vi "SetDacSafe2.vi"(1 "New Value (mV)":sgl format="%.2f", 2 "Actual Value DAC (mV)":dbl=299.98779296875 format="%.2f", 3 "DAC Nr.":i32=3 min=1 max=8 step=1) -> (0 "Voltage (mV) 2":sgl format="%.4f")   [LabVIEW 2011]
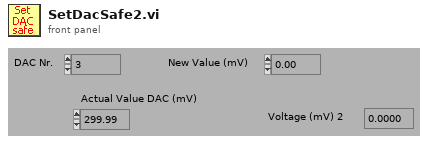
[diagram p1: front panel]
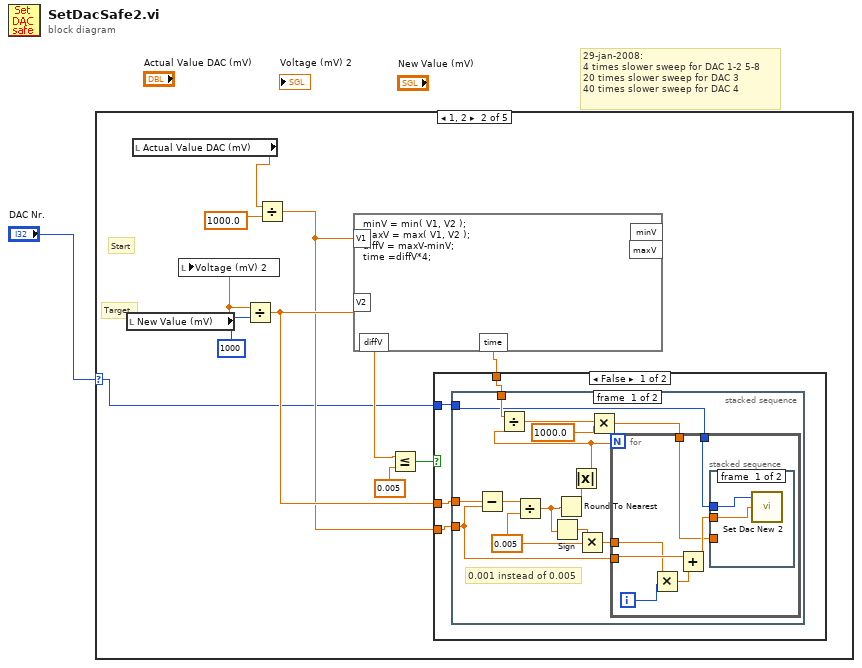
[diagram p0: block diagram]
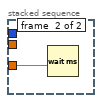
[diagram p3: hidden frame]
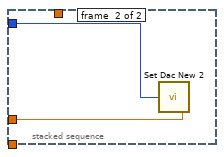
[diagram p4: hidden frame]
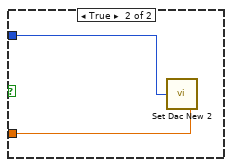
[diagram p5: hidden frame]
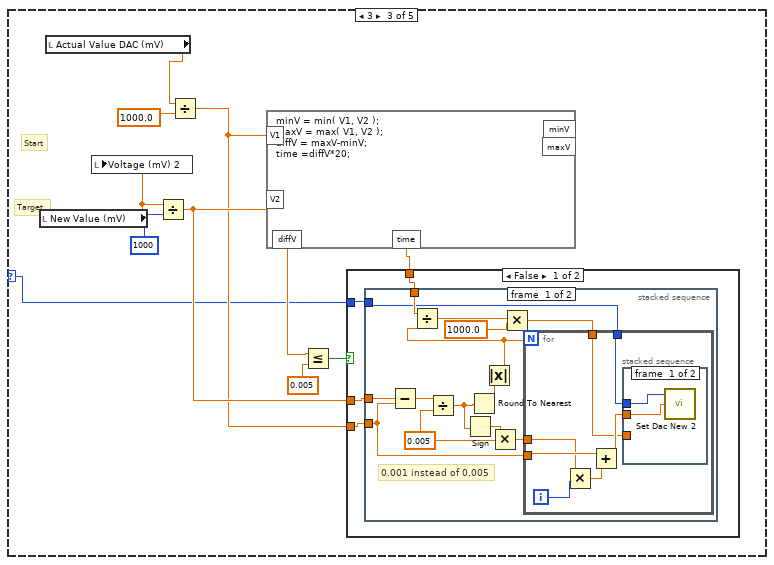
[diagram p6: hidden frame]
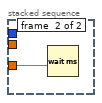
[diagram p7: hidden frame]
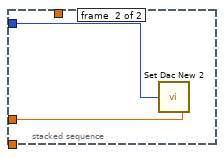
[diagram p8: hidden frame]
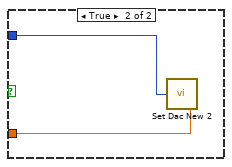
[diagram p9: hidden frame]
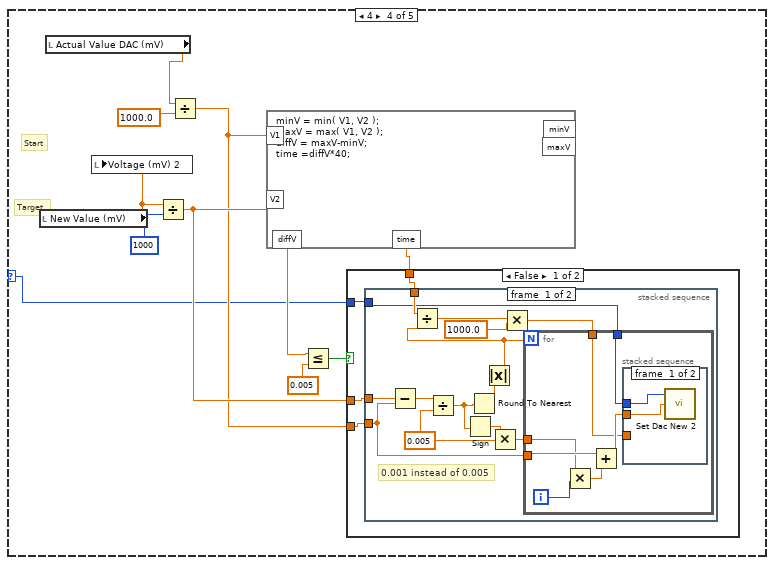
[diagram p10: hidden frame]
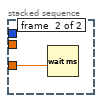
[diagram p11: hidden frame]
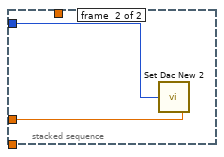
[diagram p12: hidden frame]
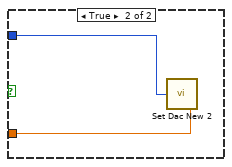
[diagram p13: hidden frame]
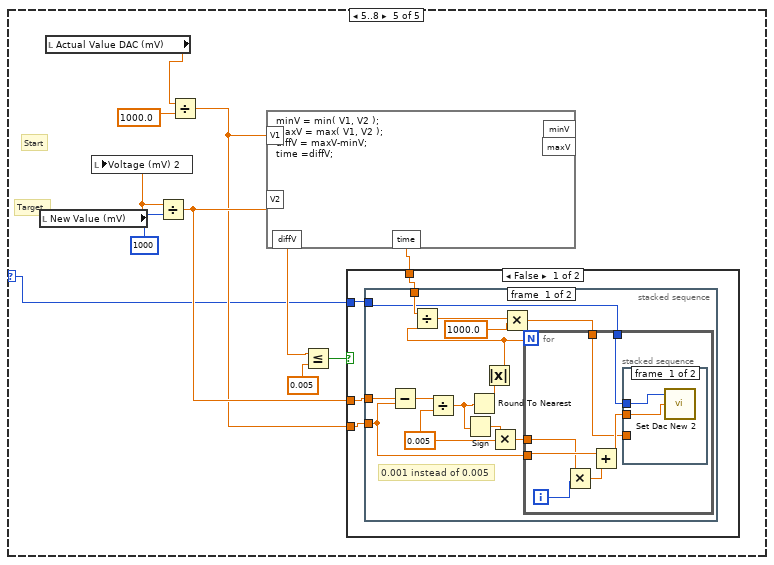
[diagram p14: hidden frame]
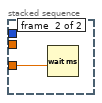
[diagram p15: hidden frame]
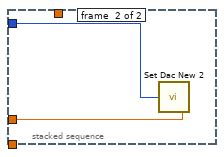
[diagram p16: hidden frame]
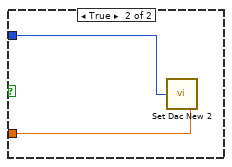
[diagram p17: hidden frame]
diagram:
  # "29-jan-2008: \n4 times slower sweep for DAC 1-2 5-8\n20 times slower sweep for DAC 3\n40 times slower sweep for DAC 4"
  n1 = case shown="1, 2" "DAC Nr." {
    selector: "DAC Nr." -> [_ w2 w45 w88 w131]
    frame 0, Default {
    }
    frame 1, 2 {
      # "Target"
      # "Start"
      n2 = local read "New Value (mV)"() -> (w3:sgl)
      n3 = local read "Actual Value DAC (mV)"() -> (w4:dbl)
      n4 = local write "Voltage (mV) 2"(w3) -> ()
      n5 = Divide(x=w3, y=1000) -> (x/y=w11:sgl)
      n6 = Divide(x=w4, y=1000.0) -> (x/y=w6:dbl)
      n7 = formula code="minV = min( V1, V2 );\nmaxV = max( V1, V2 );\ndiffV = maxV-minV;\ntime =diffV*4;"("V1"=w6, "V2"=w11) -> ("time"=w10:dbl, "diffV"=w9:dbl)  [unwired: 2 out]
      n8 = Less Or Equal?(x=w9, y=0.005) -> (x <= y?=w7:bool)
      n9 = case shown="False" w7 {
        tunnel: w6 -> [w15 _]
        tunnel: w11 -> [w16 w43]
        tunnel: w2 -> [w14 w44]
        tunnel: w10 -> [w13 _]
        frame False {
          n10 = stacked-sequence {
            tunnel: w16 -> [w30 w42]
            tunnel: w15 -> [w27 _]
            tunnel: w14 -> [w17 w41]
            tunnel: w13 -> [w25 _]
            frame #0 {
              w28 = 0.005 ("y")
              # "0.001 instead of 0.005"
              n11 = Subtract(x=w30, y=w27) -> (x-y=w29:dbl)
              n12 = Divide(x=w29, y=w28) -> (x/y=w20:dbl)
              n13 = Sign(1:w20) -> (0:w19:dbl)
              n14 = Round To Nearest(number=w20) -> (nearest integer value=w26:dbl)
              n15 = Absolute Value(x=w26) -> (abs(x)=w21:dbl)
              n16 = Divide(x=w25, y=w21) -> (x/y=w24:dbl)
              n17 = Multiply(x=w19, y=w28) -> (x*y=w18:dbl)
              n18 = Multiply(x=w24, y=1000.0) -> (x*y=w22:dbl)
              n19 = for {
                N: w21 -> [_]
                tunnel: w27 -> [w36]
                tunnel: w17 -> [w33]
                tunnel: w22 -> [w32]
                tunnel: w18 -> [w31]
                i -> [w37]
                n20 = Multiply(x=w31, y=w37) -> (x*y=w35:dbl)
                n21 = Add(x=w36, y=w35) -> (x+y=w34:dbl)
                n22 = stacked-sequence {
                  tunnel: w34 -> [w39 _]
                  tunnel: w33 -> [w38 _]
                  tunnel: w32 -> [_ w40]
                  frame #0 {
                    n23 = call "Set Dac New 2.vi"("DATA (V)"=w39, "DAC nr"=w38) -> ()
                  }
                  frame #1 {
                    n24 = Wait (ms)(milliseconds to wait=w40) -> ()  [unwired: 1 out]
                  }
                }
              }
            }
            frame #1 {
              n25 = call "Set Dac New 2.vi"("DATA (V)"=w42, "DAC nr"=w41) -> ()
            }
          }
        }
        frame True {
          n26 = call "Set Dac New 2.vi"("DATA (V)"=w43, "DAC nr"=w44) -> ()
        }
      }
    }
    frame 3 {
      # "20  times slower for DAC 3 driving top gates"
      # "Target"
      # "Start"
      n27 = local read "New Value (mV)"() -> (w46:sgl)
      n28 = local read "Actual Value DAC (mV)"() -> (w47:dbl)
      n29 = local write "Voltage (mV) 2"(w46) -> ()
      n30 = Divide(x=w46, y=1000) -> (x/y=w54:sgl)
      n31 = Divide(x=w47, y=1000.0) -> (x/y=w49:dbl)
      n32 = formula code="minV = min( V1, V2 );\nmaxV = max( V1, V2 );\ndiffV = maxV-minV;\ntime =diffV*20;"("V1"=w49, "V2"=w54) -> ("time"=w53:dbl, "diffV"=w52:dbl)  [unwired: 2 out]
      n33 = Less Or Equal?(x=w52, y=0.005) -> (x <= y?=w50:bool)
      n34 = case shown="False" w50 {
        tunnel: w49 -> [w58 _]
        tunnel: w54 -> [w59 w86]
        tunnel: w45 -> [w57 w87]
        tunnel: w53 -> [w56 _]
        frame False {
          n35 = stacked-sequence {
            tunnel: w59 -> [w73 w85]
            tunnel: w58 -> [w70 _]
            tunnel: w57 -> [w60 w84]
            tunnel: w56 -> [w68 _]
            frame #0 {
              w71 = 0.005 ("y")
              # "0.001 instead of 0.005"
              n36 = Subtract(x=w73, y=w70) -> (x-y=w72:dbl)
              n37 = Divide(x=w72, y=w71) -> (x/y=w63:dbl)
              n38 = Sign(1:w63) -> (0:w62:dbl)
              n39 = Round To Nearest(number=w63) -> (nearest integer value=w69:dbl)
              n40 = Absolute Value(x=w69) -> (abs(x)=w64:dbl)
              n41 = Divide(x=w68, y=w64) -> (x/y=w67:dbl)
              n42 = Multiply(x=w62, y=w71) -> (x*y=w61:dbl)
              n43 = Multiply(x=w67, y=1000.0) -> (x*y=w65:dbl)
              n44 = for {
                N: w64 -> [_]
                tunnel: w70 -> [w79]
                tunnel: w60 -> [w76]
                tunnel: w65 -> [w75]
                tunnel: w61 -> [w74]
                i -> [w80]
                n45 = Multiply(x=w74, y=w80) -> (x*y=w78:dbl)
                n46 = Add(x=w79, y=w78) -> (x+y=w77:dbl)
                n47 = stacked-sequence {
                  tunnel: w77 -> [w82 _]
                  tunnel: w76 -> [w81 _]
                  tunnel: w75 -> [_ w83]
                  frame #0 {
                    n48 = call "Set Dac New 2.vi"("DATA (V)"=w82, "DAC nr"=w81) -> ()
                  }
                  frame #1 {
                    n49 = Wait (ms)(milliseconds to wait=w83) -> ()  [unwired: 1 out]
                  }
                }
              }
            }
            frame #1 {
              n50 = call "Set Dac New 2.vi"("DATA (V)"=w85, "DAC nr"=w84) -> ()
            }
          }
        }
        frame True {
          n51 = call "Set Dac New 2.vi"("DATA (V)"=w86, "DAC nr"=w87) -> ()
        }
      }
    }
    frame 4 {
      # "40 times slower for DAC 4 driving HV"
      # "Target"
      # "Start"
      n52 = local read "New Value (mV)"() -> (w89:sgl)
      n53 = local read "Actual Value DAC (mV)"() -> (w90:dbl)
      n54 = local write "Voltage (mV) 2"(w89) -> ()
      n55 = Divide(x=w89, y=1000) -> (x/y=w97:sgl)
      n56 = Divide(x=w90, y=1000.0) -> (x/y=w92:dbl)
      n57 = formula code="minV = min( V1, V2 );\nmaxV = max( V1, V2 );\ndiffV = maxV-minV;\ntime =diffV*40;"("V1"=w92, "V2"=w97) -> ("time"=w96:dbl, "diffV"=w95:dbl)  [unwired: 2 out]
      n58 = Less Or Equal?(x=w95, y=0.005) -> (x <= y?=w93:bool)
      n59 = case shown="False" w93 {
        tunnel: w92 -> [w101 _]
        tunnel: w97 -> [w102 w129]
        tunnel: w88 -> [w100 w130]
        tunnel: w96 -> [w99 _]
        frame False {
          n60 = stacked-sequence {
            tunnel: w102 -> [w116 w128]
            tunnel: w101 -> [w113 _]
            tunnel: w100 -> [w103 w127]
            tunnel: w99 -> [w111 _]
            frame #0 {
              w114 = 0.005 ("y")
              # "0.001 instead of 0.005"
              n61 = Subtract(x=w116, y=w113) -> (x-y=w115:dbl)
              n62 = Divide(x=w115, y=w114) -> (x/y=w106:dbl)
              n63 = Sign(1:w106) -> (0:w105:dbl)
              n64 = Round To Nearest(number=w106) -> (nearest integer value=w112:dbl)
              n65 = Absolute Value(x=w112) -> (abs(x)=w107:dbl)
              n66 = Divide(x=w111, y=w107) -> (x/y=w110:dbl)
              n67 = Multiply(x=w105, y=w114) -> (x*y=w104:dbl)
              n68 = Multiply(x=w110, y=1000.0) -> (x*y=w108:dbl)
              n69 = for {
                N: w107 -> [_]
                tunnel: w113 -> [w122]
                tunnel: w103 -> [w119]
                tunnel: w108 -> [w118]
                tunnel: w104 -> [w117]
                i -> [w123]
                n70 = Multiply(x=w117, y=w123) -> (x*y=w121:dbl)
                n71 = Add(x=w122, y=w121) -> (x+y=w120:dbl)
                n72 = stacked-sequence {
                  tunnel: w120 -> [w125 _]
                  tunnel: w119 -> [w124 _]
                  tunnel: w118 -> [_ w126]
                  frame #0 {
                    n73 = call "Set Dac New 2.vi"("DATA (V)"=w125, "DAC nr"=w124) -> ()
                  }
                  frame #1 {
                    n74 = Wait (ms)(milliseconds to wait=w126) -> ()  [unwired: 1 out]
                  }
                }
              }
            }
            frame #1 {
              n75 = call "Set Dac New 2.vi"("DATA (V)"=w128, "DAC nr"=w127) -> ()
            }
          }
        }
        frame True {
          n76 = call "Set Dac New 2.vi"("DATA (V)"=w129, "DAC nr"=w130) -> ()
        }
      }
    }
    frame 5..8 {
      # "Target"
      # "Start"
      n77 = local read "New Value (mV)"() -> (w132:sgl)
      n78 = local read "Actual Value DAC (mV)"() -> (w133:dbl)
      n79 = local write "Voltage (mV) 2"(w132) -> ()
      n80 = Divide(x=w132, y=1000) -> (x/y=w140:sgl)
      n81 = Divide(x=w133, y=1000.0) -> (x/y=w135:dbl)
      n82 = formula code="minV = min( V1, V2 );\nmaxV = max( V1, V2 );\ndiffV = maxV-minV;\ntime =diffV;"("V1"=w135, "V2"=w140) -> ("time"=w139:dbl, "diffV"=w138:dbl)  [unwired: 2 out]
      n83 = Less Or Equal?(x=w138, y=0.005) -> (x <= y?=w136:bool)
      n84 = case shown="False" w136 {
        tunnel: w135 -> [w144 _]
        tunnel: w140 -> [w145 w172]
        tunnel: w131 -> [w143 w173]
        tunnel: w139 -> [w142 _]
        frame False {
          n85 = stacked-sequence {
            tunnel: w145 -> [w159 w171]
            tunnel: w144 -> [w156 _]
            tunnel: w143 -> [w146 w170]
            tunnel: w142 -> [w154 _]
            frame #0 {
              w157 = 0.005 ("y")
              # "0.001 instead of 0.005"
              n86 = Subtract(x=w159, y=w156) -> (x-y=w158:dbl)
              n87 = Divide(x=w158, y=w157) -> (x/y=w149:dbl)
              n88 = Sign(1:w149) -> (0:w148:dbl)
              n89 = Round To Nearest(number=w149) -> (nearest integer value=w155:dbl)
              n90 = Absolute Value(x=w155) -> (abs(x)=w150:dbl)
              n91 = Divide(x=w154, y=w150) -> (x/y=w153:dbl)
              n92 = Multiply(x=w148, y=w157) -> (x*y=w147:dbl)
              n93 = Multiply(x=w153, y=1000.0) -> (x*y=w151:dbl)
              n94 = for {
                N: w150 -> [_]
                tunnel: w156 -> [w165]
                tunnel: w146 -> [w162]
                tunnel: w151 -> [w161]
                tunnel: w147 -> [w160]
                i -> [w166]
                n95 = Multiply(x=w160, y=w166) -> (x*y=w164:dbl)
                n96 = Add(x=w165, y=w164) -> (x+y=w163:dbl)
                n97 = stacked-sequence {
                  tunnel: w163 -> [w168 _]
                  tunnel: w162 -> [w167 _]
                  tunnel: w161 -> [_ w169]
                  frame #0 {
                    n98 = call "Set Dac New 2.vi"("DATA (V)"=w168, "DAC nr"=w167) -> ()
                  }
                  frame #1 {
                    n99 = Wait (ms)(milliseconds to wait=w169) -> ()  [unwired: 1 out]
                  }
                }
              }
            }
            frame #1 {
              n100 = call "Set Dac New 2.vi"("DATA (V)"=w171, "DAC nr"=w170) -> ()
            }
          }
        }
        frame True {
          n101 = call "Set Dac New 2.vi"("DATA (V)"=w172, "DAC nr"=w173) -> ()
        }
      }
    }
  }
